vi "Calculate Direction.vi"(8 "Y1":dbl=-121.824251 format="%#_14g", 9 "Y0":dbl format="%#_11g", 10 "X1":dbl=39.689375 format="%#_14g", 11 "X0":dbl format="%#_11g") -> (0 "Error":bool, 1 "Delta X":dbl format="%#_11g", 2 "Delta Y":dbl format="%#_10g", 3 "Destination Bearing":dbl)   [LabVIEW 2011]
panel:
  out "Direction":string
  out "XY Graph":cluster{"Array":dbl[], "Array 2":dbl[]}(graph)
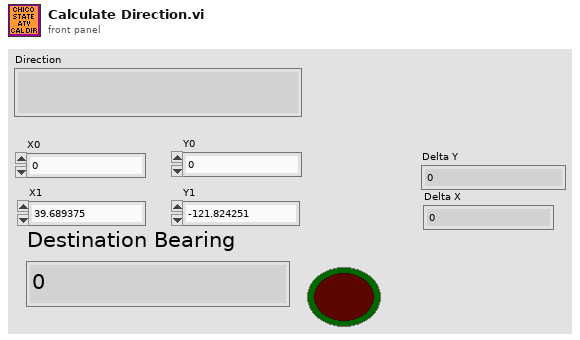
[diagram p1: front panel]
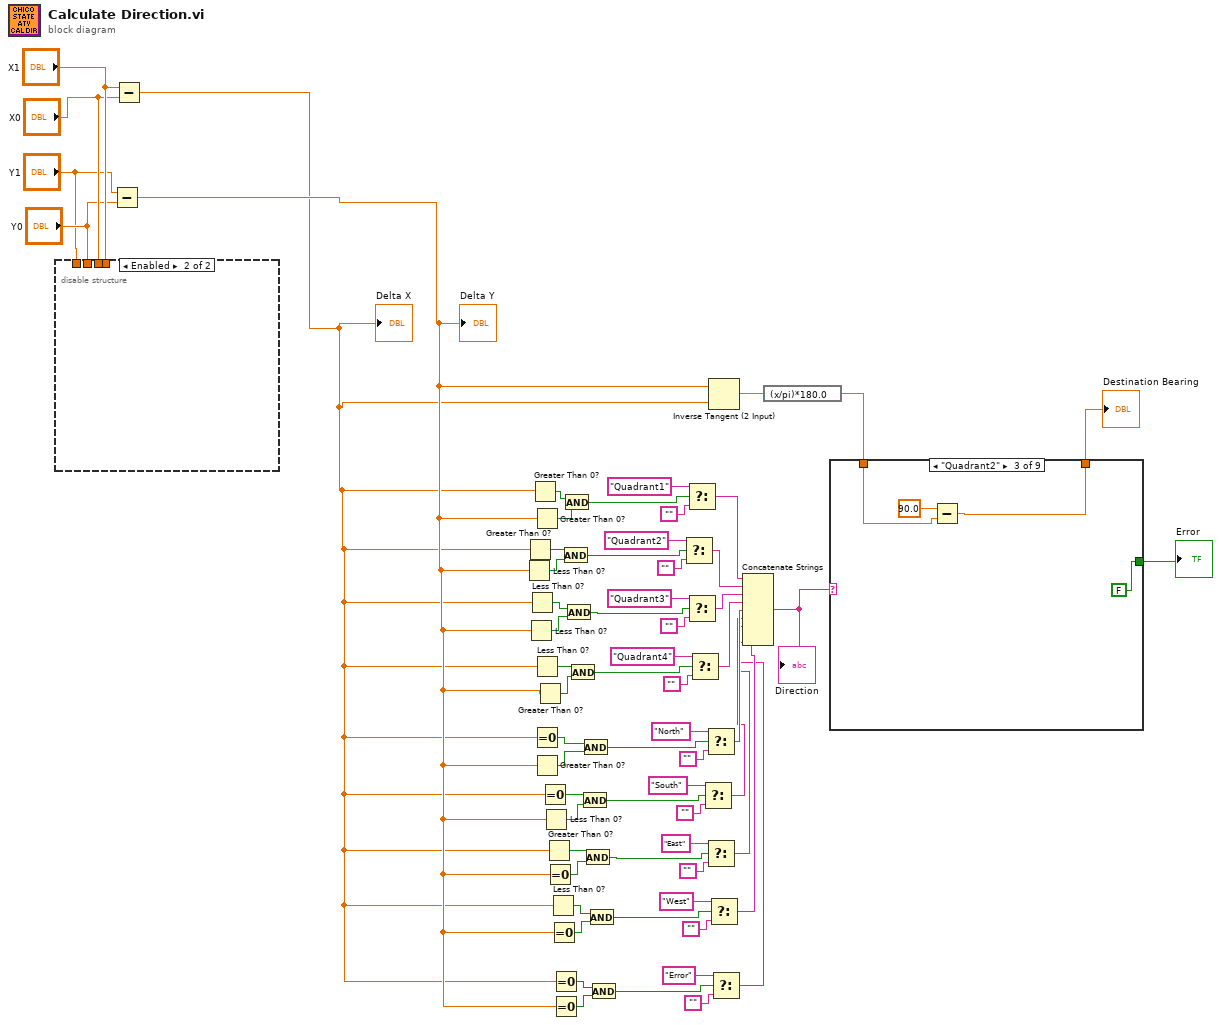
[diagram p0: block diagram]
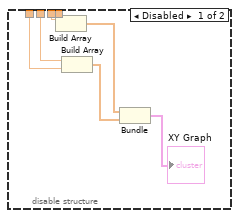
[diagram p2: hidden frame]
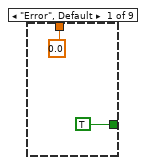
[diagram p3: hidden frame]
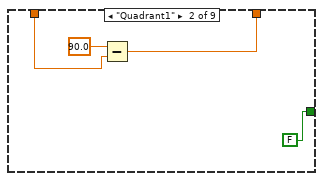
[diagram p4: hidden frame]
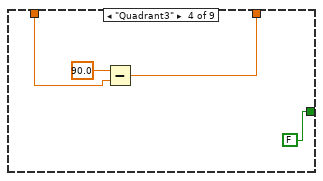
[diagram p5: hidden frame]
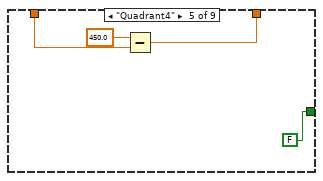
[diagram p6: hidden frame]
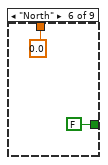
[diagram p7: hidden frame]
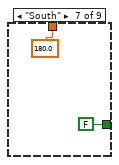
[diagram p8: hidden frame]
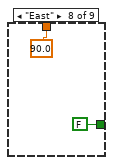
[diagram p9: hidden frame]
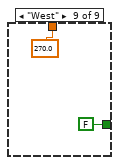
[diagram p10: hidden frame]
diagram:
  n1 = disable-structure shown="Enabled" {
    disable-tunnel: "X1" -> [w71 _]
    disable-tunnel: "X0" -> [w70 _]
    disable-tunnel: "Y0" -> [w69 _]
    disable-tunnel: "Y1" -> [w68 _]
    frame Disabled {
      n2 = Build Array(w70, w71) -> (w67:dbl[])
      n3 = Build Array(w69, w68) -> (w66:dbl[])
      n4 = Bundle(w67, w66) -> (→"XY Graph":cluster{dbl[], dbl[]})  [unwired: 1 in]
    }
    frame Enabled {
    }
  }
  n5 = Subtract(x="Y1", y="Y0") -> (x-y=w2:dbl)
  "Delta Y" <- w2
  n6 = Subtract(x="X1", y="X0") -> (x-y=w1:dbl)
  "Delta X" <- w1
  n7 = Less Than 0?(x=w2) -> (x < 0?=w57:bool)
  n8 = Greater Than 0?(x=w1) -> (x > 0?=w11:bool)
  n9 = Less Than 0?(x=w2) -> (x < 0?=w47:bool)
  n10 = Less Than 0?(x=w1) -> (x < 0?=w48:bool)
  n11 = Greater Than 0?(x=w1) -> (x > 0?=w13:bool)
  n12 = Greater Than 0?(x=w2) -> (x > 0?=w12:bool)
  n13 = Less Than 0?(x=w1) -> (x < 0?=w46:bool)
  n14 = Equal To 0?(x=w1) -> (x = 0?=w21:bool)
  n15 = Greater Than 0?(x=w2) -> (x > 0?=w20:bool)
  n16 = Greater Than 0?(x=w2) -> (x > 0?=w10:bool)
  n17 = Equal To 0?(x=w1) -> (x = 0?=w19:bool)
  n18 = Less Than 0?(x=w2) -> (x < 0?=w18:bool)
  n19 = Greater Than 0?(x=w1) -> (x > 0?=w17:bool)
  n20 = Equal To 0?(x=w2) -> (x = 0?=w16:bool)
  n21 = Less Than 0?(x=w1) -> (x < 0?=w14:bool)
  n22 = Equal To 0?(x=w2) -> (x = 0?=w15:bool)
  n23 = Equal To 0?(x=w1) -> (x = 0?=w4:bool)
  n24 = Equal To 0?(x=w2) -> (x = 0?=w9:bool)
  n25 = And(x=w11, y=w57) -> (x .and. y?=w56:bool)
  n26 = And(x=w13, y=w12) -> (x .and. y?=w55:bool)
  n27 = And(x=w48, y=w47) -> (x .and. y?=w54:bool)
  n28 = And(x=w46, y=w10) -> (x .and. y?=w53:bool)
  n29 = And(x=w19, y=w18) -> (x .and. y?=w34:bool)
  n30 = And(x=w21, y=w20) -> (x .and. y?=w35:bool)
  n31 = And(x=w17, y=w16) -> (x .and. y?=w36:bool)
  n32 = And(x=w14, y=w15) -> (x .and. y?=w37:bool)
  n33 = And(x=w4, y=w9) -> (x .and. y?=w6:bool)
  n34 = Select(t="Quadrant2", s=w56, f="") -> (s? t:f=w49:string)
  n35 = Select(t="Quadrant1", s=w55, f="") -> (s? t:f=w52:string)
  n36 = Select(t="Quadrant3", s=w54, f="") -> (s? t:f=w50:string)
  n37 = Select(t="Quadrant4", s=w53, f="") -> (s? t:f=w51:string)
  n38 = Select(t="South", s=w34, f="") -> (s? t:f=w24:string)
  n39 = Select(t="North", s=w35, f="") -> (s? t:f=w25:string)
  n40 = Select(t="East", s=w36, f="") -> (s? t:f=w23:string)
  n41 = Inverse Tangent (2 Input)(1:w1, 2:w2) -> (0:w39:dbl)
  n42 = Select(t="West", s=w37, f="") -> (s? t:f=w22:string)
  n43 = Select(t="Error", s=w6, f="") -> (s? t:f=w5:string)
  n44 = Concatenate Strings(w52, w49, w50, w51, w25, w24, w23, w22, w5) -> (w45:string)
  "Direction" <- w45
  n45 = expression code="(x/pi)*180.0" ("radians to degrees")(w39) -> (w38:dbl)
  n46 = case shown="\"Quadrant2\"" w45 {
    tunnel: [0.0 w76 w80 w83 w89 0.0 180.0 90.0 270.0] -> w40
    tunnel: w38 -> [_ w75 w79 w84 w88 _ _ _ _]
    tunnel: [TRUE ("Error") FALSE FALSE FALSE FALSE FALSE ("Error") FALSE ("Error") FALSE ("Error") FALSE ("Error")] -> w3
    frame "Error", Default {
    }
    frame "Quadrant1" {
      n47 = Subtract(x=90.0, y=w75) -> (x-y=w76:dbl)
    }
    frame "Quadrant2" {
      n48 = Subtract(x=90.0, y=w79) -> (x-y=w80:dbl)
    }
    frame "Quadrant3" {
      n49 = Subtract(x=90.0, y=w84) -> (x-y=w83:dbl)
    }
    frame "Quadrant4" {
      n50 = Subtract(x=450.0, y=w88) -> (x-y=w89:dbl)
    }
    frame "North" {
    }
    frame "South" {
    }
    frame "East" {
    }
    frame "West" {
    }
  }
  "Error" <- w3
  "Destination Bearing" <- w40
